vi "ProgrammWithEventAndStateMachine.vi"() -> ()   [LabVIEW 2020]
uses:
  #typedef_States.ctl
  #typedef_Database.ctl
  <vilib>/picture/picture.llb/imagedata.ctl
  <vilib>/event_ctls.llb/eventvkey.ctl
  shell32.dll
panel:
  in  "EndOfProgram":bool
  in  "BROWSEINFO 2":T1={"hWndOwner"=0, "pidlRoot"=0, "pszDisplayName"=0, "lpszTitle"=0, "ulFlags"=1, "lpfn"=0, "lParam"=0, "iImage"=0}
  in  "List of images":i32[](listbox)
  in  "Path":string
  out "2D Picture":picture
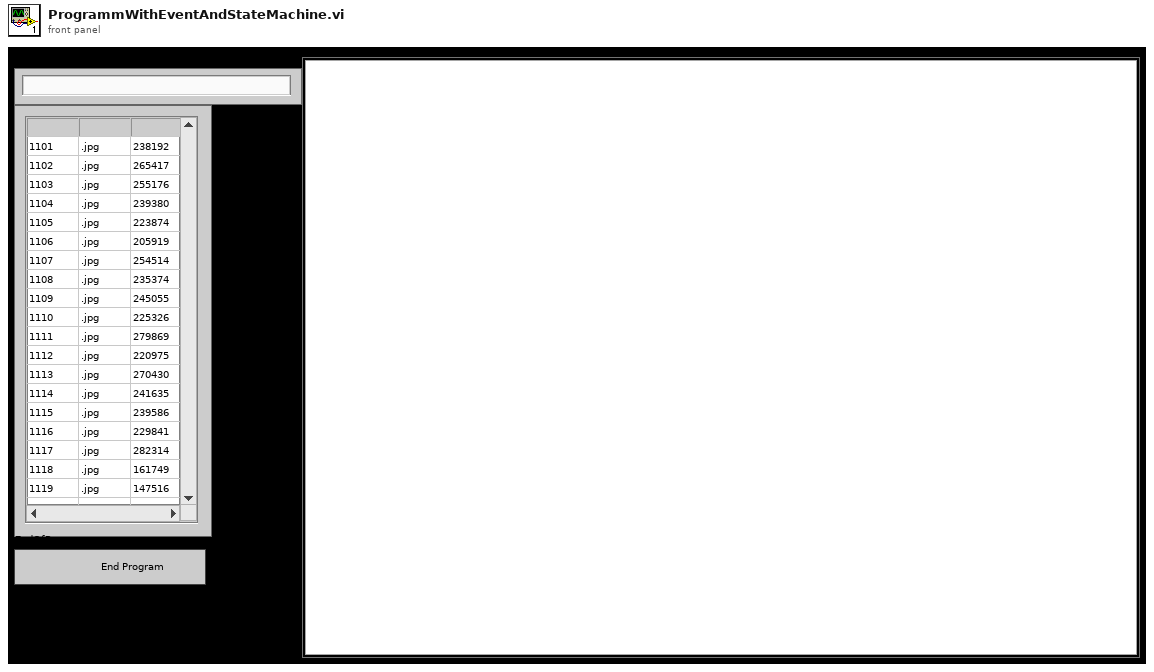
[diagram p1: front panel]
types:
  T1 = cluster{"hWndOwner":i32, "pidlRoot":i32, "pszDisplayName":i32, "lpszTitle":i32, "ulFlags":i32, "lpfn":i32, "lParam":i32, "iImage":i32}
  T2 = typedef "#typedef_States.ctl" = enum16{"Initialize", "CheckButton", "OpenFromKey", "OpenFromPath", "ImageView", "AreaOfImageResize", "ImageResize", "ChangeImage", "ShowNext", "ShowPrevious", "LoadImagesName", "End"}
  T3 = typedef "#typedef_Database.ctl" = cluster{"Folder Directory":string, "Name of images":string[], "PreviousState":T2, "NumberOfRow":i32, "PanelResizeMeasurement":cluster{"Right":i16, "Left":i16, "Bottom":i16, "Top":i16}, "CurrentImageData":T4, "ImageChangeKey":T5, "IsShiftPressed?":bool}
  T4 = typedef "imagedata.ctl" = cluster{"image type":i32, "image depth":i32, "image":u8[], "mask":u8[], "colors":u32[], "Rectangle":cluster{"left":i16, "top":i16, "right":i16, "bottom":i16}}
  T5 = typedef "eventvkey.ctl" = enum16{"ASCII", "Enter", "Return", "Shift", "Ctrl", "Alt", "Cmd", "Opt", "Caps", "NumLock", "Clear", "Break", "Up", "Down", "Left", "Right", "Insert", "Delete", "Home", "End", "PageUp", "PageDown", "Escape", "Help", "Pause", "ScrollLock", "F1", "F2", "F3", "F4", "F5", "F6", "F7", "F8", "F9", "F10", "F11", "F12", "F13", "F14", "F15", "F16", "F17", "F18", "F19", "F20", "F21", "F22", "F23", "F24", "Play", "VolumeUp", "VolumeDown", "Mute", "Two Byte Char"}
  T6 = cluster{"Shift":bool, "Ctrl":bool, "Alt":bool, "Cmd":bool, "Opt":bool}
  T7 = typedef "LVRectTypeDef.ctl" = cluster{"Left":i16, "Top":i16, "Right":i16, "Bottom":i16}
  T8 = typedef "LVBoundsTypeDef.ctl" = cluster{"Width":u32, "Height":u32}
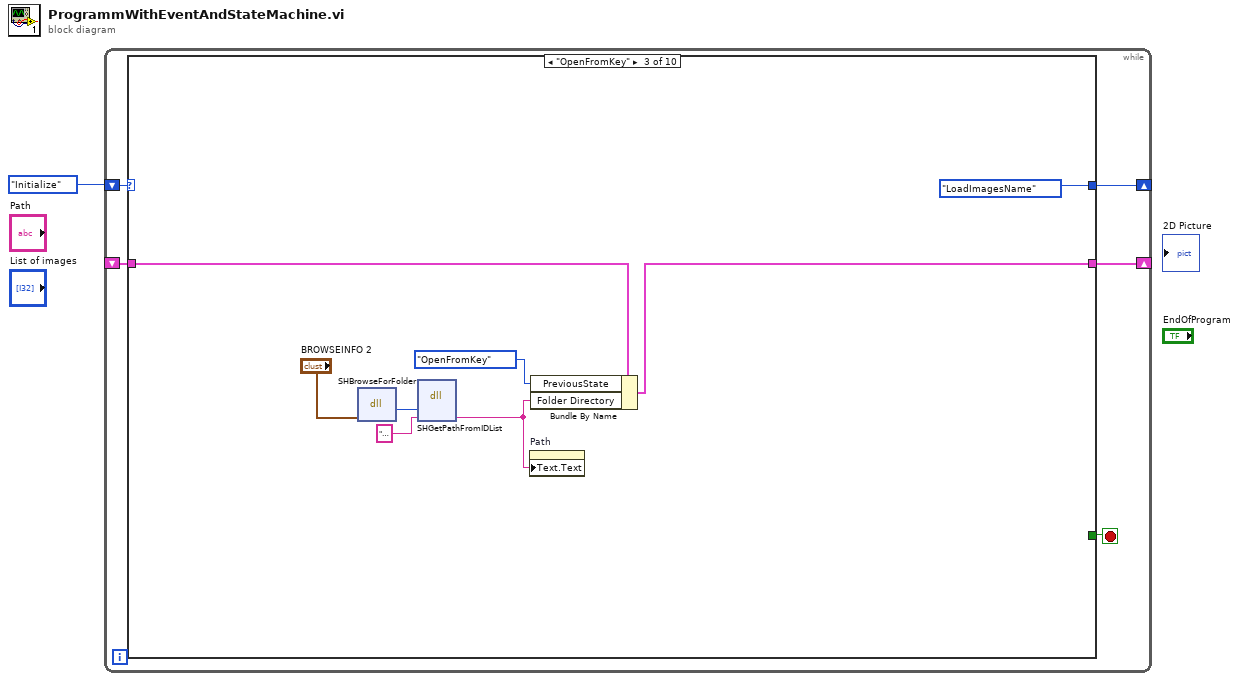
[diagram p0: block diagram]
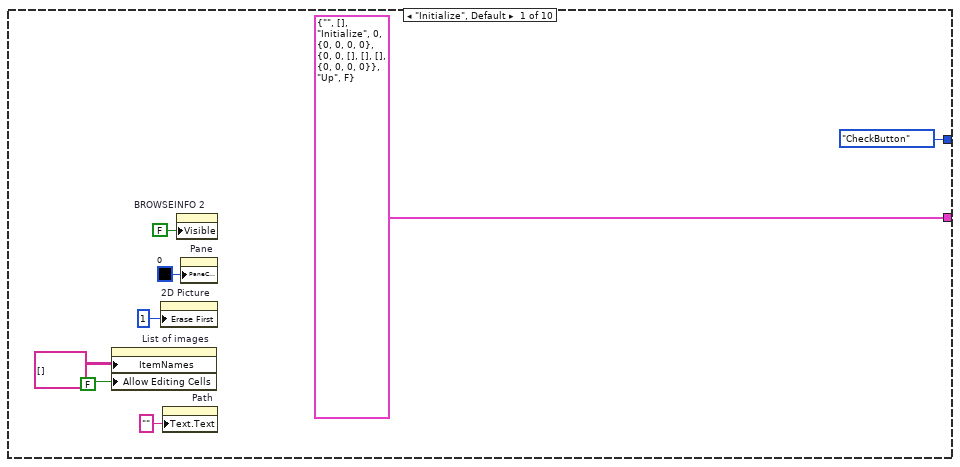
[diagram p2: hidden frame]
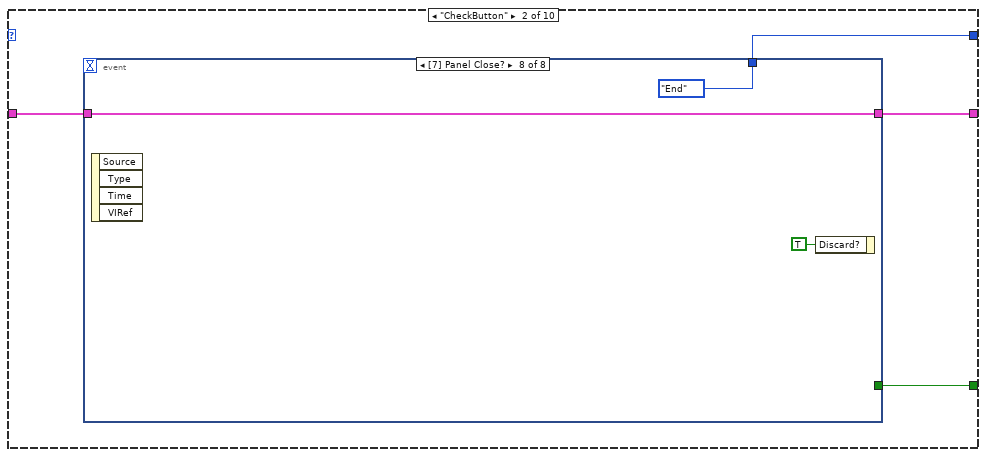
[diagram p3: hidden frame]
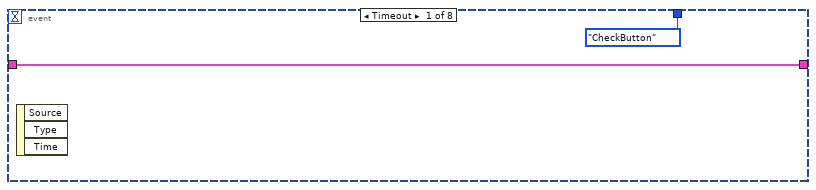
[diagram p4: hidden frame]
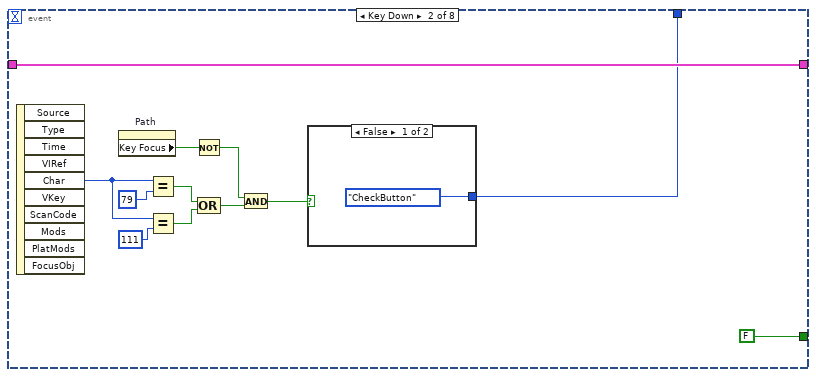
[diagram p5: hidden frame]
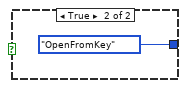
[diagram p6: hidden frame]
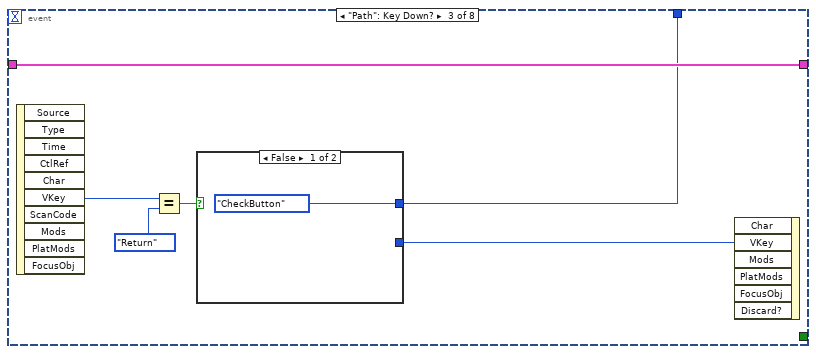
[diagram p7: hidden frame]
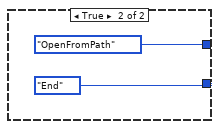
[diagram p8: hidden frame]
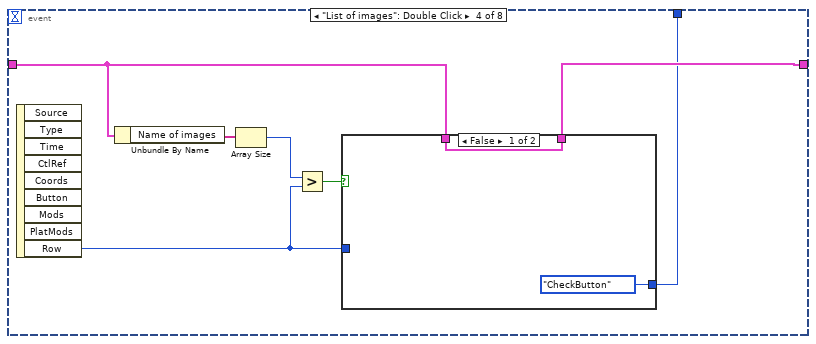
[diagram p9: hidden frame]
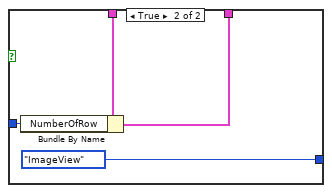
[diagram p10: hidden frame]
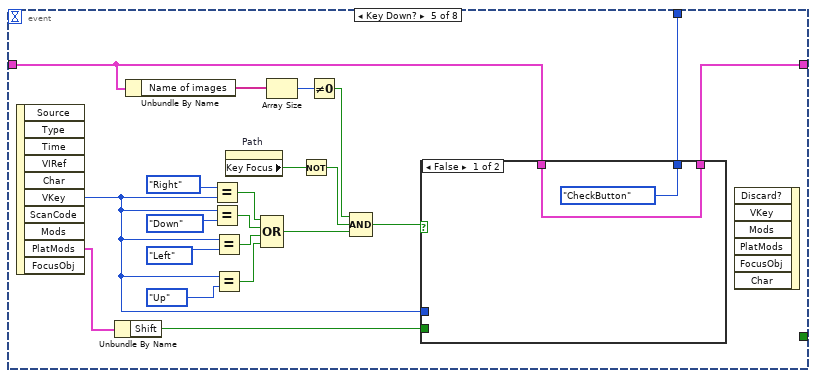
[diagram p11: hidden frame]
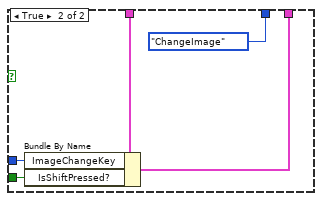
[diagram p12: hidden frame]
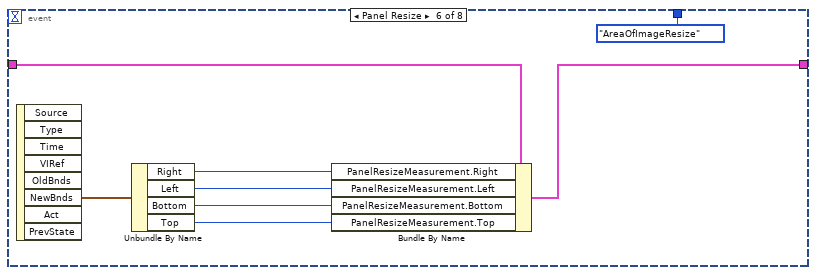
[diagram p13: hidden frame]
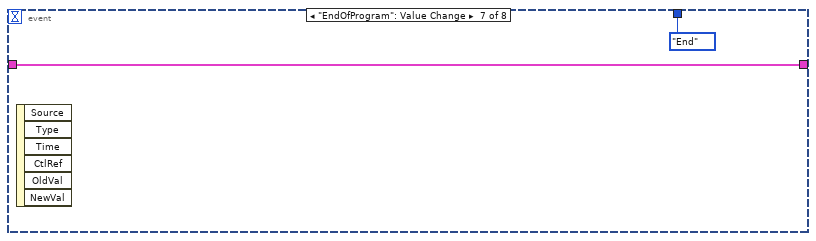
[diagram p14: hidden frame]
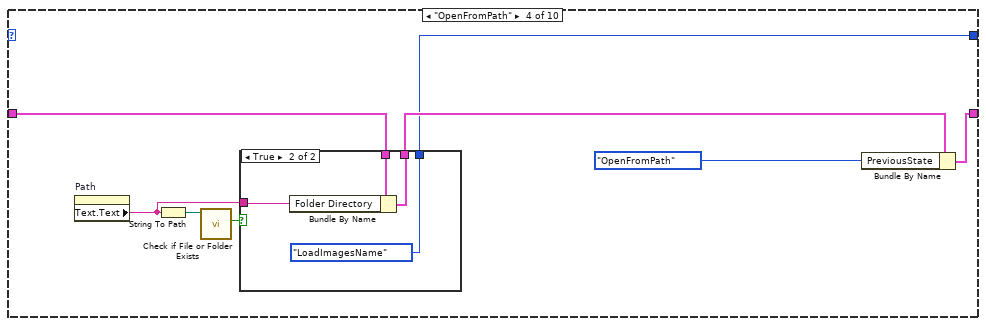
[diagram p15: hidden frame]
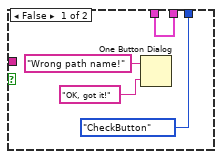
[diagram p16: hidden frame]
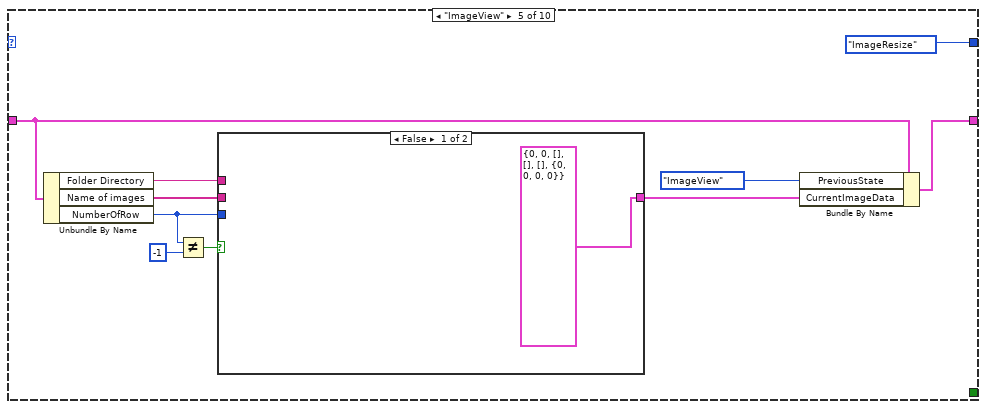
[diagram p17: hidden frame]
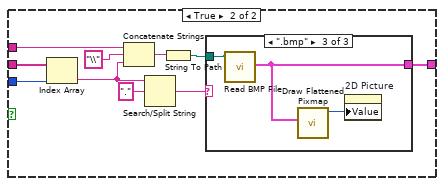
[diagram p18: hidden frame]
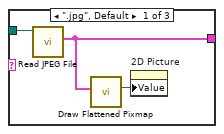
[diagram p19: hidden frame]
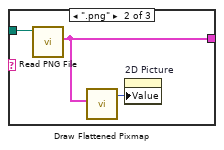
[diagram p20: hidden frame]
diagram:
  n1 = while {
    shift-right: [w2] -> _
    shift-left: _ -> [w6]
    shift-right: [w3] -> _
    shift-left: #typedef_States."Initialize" ("States") -> [w4]
    stop <- w5 stop-if-true
    n2 = case shown="\"OpenFromKey\"" w4 {
      tunnel: w6 -> [_ w18 w102 w110 w128 w155 w176 w181 w252 w273]
      tunnel: [_ w17 _ _ _ _ _ _ _ TRUE] -> w5
      tunnel: [T3 {"Folder Directory"="", "Name of images"=[], "PreviousState"=enum."Initialize", "NumberOfRow"=0, "PanelResizeMeasurement"={"Right"=0, "Left"=0, "Bottom"=0, "Top"=0}, "CurrentImageData"={"image type"=0, "image depth"=0, "image"=[], "mask"=[], "colors"=[], "Rectangle"={"left"=0, "top"=0, "right"=0, "bottom"=0}}, "ImageChangeKey"=enum."Up", "IsShiftPressed?"=FALSE} ("Database") w16 w101 w108 w127 w154 w174 w183 w258 w273] -> w2
      tunnel: [#typedef_States."CheckButton" ("States") w15 #typedef_States."LoadImagesName" ("States") w106 #typedef_States."ImageResize" ("States") #typedef_States."ImageResize" ("States") #typedef_States."CheckButton" ("States") #typedef_States."ImageView" ("States") #typedef_States."ImageView" ("States") #typedef_States."End" ("States")] -> w3
      frame "Initialize", Default {
        n3 = property on="List of images" class="MCListbox (strict)"("ItemNames"=string[][] [] ("Item Names"), "Allow Editing Cells"=FALSE) -> ()  [unwired: 2 in, 2 out]
        n4 = property on="2D Picture" class="Pict"("Erase First"=u8 1) -> ()  [unwired: 2 in, 2 out]
        n5 = property on="Path" class="Str"("Text.Text"="") -> ()  [unwired: 2 in, 2 out]
        n6 = property on="BROWSEINFO 2" class="Clust (strict)"("Visible"=FALSE) -> ()  [unwired: 2 in, 2 out]
        n7 = property on="Pane" class="Pane"("PaneColor"=u32 0 ("Pane Color")) -> ()  [unwired: 2 in, 2 out]
      }
      frame "CheckButton" {
        n8 = event shown="[7] Panel Close?" {
          selector: _ -> [_ _ _ _ _ _ _ _]
          dyn-events: _ -> [_ _ _ _ _ _ _ _]
          timeout: _ -> [_ _ _ _ _ _ _ _]
          tunnel: w18 -> [w20 w22 w36 w49 w65 w91 w94 w95]
          tunnel: [w20 w22 w36 w50 w66 w90 w94 w95] -> w16
          tunnel: [_ FALSE _ _ _ _ _ _] -> w17
          tunnel: [#typedef_States."CheckButton" ("States") w21 w35 w47 w67 #typedef_States."AreaOfImageResize" ("States") #typedef_States."End" ("States") #typedef_States."End" ("States")] -> w15
          event Timeout {
            n9 = event-data() -> ()  [unwired: 1 in, 3 out]
          }
          event Key Down {
            n10 = event-data() -> ("Char"=w32:i16)  [unwired: 1 in, 9 out]
            n11 = property on="Path" class="Str"() -> ("Key Focus"=w26:bool)  [unwired: 2 in, 2 out]
            n12 = Equal?(x=w32, y=i16 79) -> (x = y?=w29:bool)
            n13 = Equal?(x=w32, y=i16 111) -> (x = y?=w28:bool)
            n14 = Not(x=w26) -> (.not. x?=w25:bool)
            n15 = Compound Arithmetic op=OR(w29, w28) -> (w24:bool)
            n16 = And(x=w25, y=w24) -> (x .and. y?=w23:bool)
            n17 = case shown="False" w23 {
              tunnel: [#typedef_States."CheckButton" ("States") #typedef_States."OpenFromKey" ("States")] -> w21
              frame False {
              }
              frame True {
              }
            }
          }
          event "Path": Key Down? {
            n18 = event-data() -> ("VKey"=w39:T5)  [unwired: 1 in, 9 out]
            n19 = Equal?(x=w39, y=eventvkey."Return") -> (x = y?=w40:bool)
            n20 = case shown="False" w40 {
              tunnel: [_ eventvkey."End" ("VKey")] -> w37
              tunnel: [#typedef_States."CheckButton" ("States") #typedef_States."OpenFromPath" ("States")] -> w35
              frame False {
              }
              frame True {
              }
            }
            n21 = event-data("VKey"=w37) -> ()  [unwired: 6 in, 1 out]
          }
          event "List of images": Double Click {
            n22 = event-data() -> ("Row"=w46:i32)  [unwired: 1 in, 8 out]
            n23 = Unbundle By Name(w49) -> ("Name of images"=w48:string[])
            n24 = Array Size(array=w48) -> (size(s)=w44:i32)
            n25 = Greater?(x=w44, y=w46) -> (0:w45:bool)
            n26 = case shown="False" w45 {
              tunnel: w49 -> [w52 w56]
              tunnel: [w52 w55] -> w50
              tunnel: w46 -> [_ w54]
              tunnel: [#typedef_States."CheckButton" ("States") #typedef_States."ImageView" ("States")] -> w47
              frame False {
              }
              frame True {
                n27 = Bundle By Name(cluster=w56, "NumberOfRow"=w54) -> (w55:T3)
              }
            }
          }
          event Key Down? {
            n28 = event-data() -> ("VKey"=w64:T5, "PlatMods"=w58:T6)  [unwired: 1 in, 8 out]
            n29 = Unbundle By Name(w58) -> ("Shift"=w57:bool)
            n30 = Unbundle By Name(w65) -> ("Name of images"=w77:string[])
            n31 = Equal?(x=eventvkey."Right" ("VKey"), y=w64) -> (x = y?=w76:bool)
            n32 = Equal?(x=w64, y=eventvkey."Down" ("VKey")) -> (x = y?=w75:bool)
            n33 = Equal?(x=w64, y=eventvkey."Left" ("VKey")) -> (x = y?=w69:bool)
            n34 = Equal?(x=w64, y=eventvkey."Up" ("VKey")) -> (x = y?=w68:bool)
            n35 = property on="Path" class="Str"() -> ("Key Focus"=w74:bool)  [unwired: 2 in, 2 out]
            n36 = Compound Arithmetic op=OR(w76, w75, w69, w68) -> (w62:bool)
            n37 = Array Size(array=w77) -> (size(s)=w63:i32)
            n38 = Not(x=w74) -> (.not. x?=w61:bool)
            n39 = Not Equal To 0?(x=w63) -> (x != 0?=w60:bool)
            n40 = Compound Arithmetic op=AND(w60, w61, w62) -> (w59:bool)
            n41 = case shown="False" w59 {
              tunnel: [#typedef_States."CheckButton" ("States") #typedef_States."ChangeImage" ("States")] -> w67
              tunnel: w65 -> [w78 w83]
              tunnel: [w78 w82] -> w66
              tunnel: w64 -> [_ w81]
              tunnel: w57 -> [_ w80]
              frame False {
              }
              frame True {
                n42 = Bundle By Name(cluster=w83, "ImageChangeKey"=w81, "IsShiftPressed?"=w80) -> (w82:T3)
              }
            }
            n43 = event-data() -> ()  [unwired: 7 in, 1 out]
          }
          event Panel Resize {
            n44 = event-data() -> ("NewBnds"=w89:T7)  [unwired: 1 in, 7 out]
            n45 = Unbundle By Name(w89) -> ("Right"=w88:i16, "Left"=w87:i16, "Bottom"=w86:i16, "Top"=w85:i16)
            n46 = Bundle By Name(cluster=w91, "PanelResizeMeasurement.Right"=w88, "PanelResizeMeasurement.Left"=w87, "PanelResizeMeasurement.Bottom"=w86, "PanelResizeMeasurement.Top"=w85) -> (w90:T3)
          }
          event "EndOfProgram": Value Change {
            n47 = event-data() -> ()  [unwired: 1 in, 6 out]
          }
          event Panel Close? {
            n48 = event-data() -> ()  [unwired: 1 in, 4 out]
            n49 = event-data("Discard?"=TRUE) -> ()  [unwired: 1 in, 1 out]
          }
        }
      }
      frame "OpenFromKey" {
        n50 = dll-call lib="shell32.dll" fn="SHBrowseForFolder"("BROWSEINFO"="BROWSEINFO 2") -> ("PointerToIDList"=w104:i32)  [unwired: 4 in, 2 out]
        n51 = dll-call lib="shell32.dll" fn="SHGetPathFromIDList"("PointerToIDList"=w104, "PathBuffer"="                                                                                                                                                                                                                                                                    " ("260 char string")) -> ("PathBuffer"=w98:string)  [unwired: 5 in, 2 out]
        n52 = property on="Path" class="Str"("Text.Text"=w98) -> ()  [unwired: 2 in, 2 out]
        n53 = Bundle By Name(cluster=w102, "PreviousState"=#typedef_States."OpenFromKey" ("States"), "Folder Directory"=w98) -> (w101:T3)
      }
      frame "OpenFromPath" {
        n54 = property on="Path" class="Str"() -> ("Text.Text"=w111:string)  [unwired: 2 in, 2 out]
        n55 = String To Path(string=w111) -> (path=w113:path)
        n56 = call <vilib>:"Check if File or Folder Exists.vi"("path"=w113) -> ("file or folder exists?"=w112:bool)  [unwired: 8 in, 2 out]
        n57 = case shown="True" w112 {
          tunnel: w110 -> [w117 w121]
          tunnel: w111 -> [_ w119]
          tunnel: [w117 w120] -> w109
          tunnel: [#typedef_States."CheckButton" ("States") #typedef_States."LoadImagesName" ("States")] -> w106
          frame False {
            n58 = One Button Dialog(message="Wrong path name!", button name ("OK")="OK, got it!") -> ()  [unwired: 1 out]
          }
          frame True {
            n59 = Bundle By Name(cluster=w121, "Folder Directory"=w119) -> (w120:T3)
          }
        }
        n60 = Bundle By Name(cluster=w109, "PreviousState"=#typedef_States."OpenFromPath" ("States")) -> (w108:T3)
      }
      frame "ImageView" {
        n61 = Unbundle By Name(w128) -> ("Folder Directory"=w130:string, "Name of images"=w131:string[], "NumberOfRow"=w123:i32)
        n62 = Not Equal?(x=w123, y=-1) -> (x != y?=w124:bool)
        n63 = case shown="False" w124 {
          tunnel: w131 -> [_ w142]
          tunnel: w130 -> [_ w141]
          tunnel: w123 -> [_ w134]
          tunnel: [T4 {"image type"=0, "image depth"=0, "image"=[], "mask"=[], "colors"=[], "Rectangle"={"left"=0, "top"=0, "right"=0, "bottom"=0}} ("CurrentImageData") w133] -> w125
          frame False {
          }
          frame True {
            n64 = Index Array(array=w142, index=w134) -> (element=w139:string)
            n65 = Concatenate Strings(w141, "\\" ("string"), w139) -> (w140:string)
            n66 = Search/Split String(string=w139, search string/char (-)=".") -> (match + rest of string=w138:string)  [unwired: 1 in, 2 out]
            n67 = String To Path(string=w140) -> (path=w137:path)
            n68 = case shown="\".bmp\"" w138 {
              tunnel: w137 -> [w145 w147 w150]
              tunnel: [w143 w146 w149] -> w133
              frame ".jpg", Default {
                n69 = call <vilib>:"Read JPEG File.vi"("path to JPEG file"=w145) -> ("image data"=w143:T4)  [unwired: 8 in, 2 out]
                n70 = call <vilib>:"Draw Flattened Pixmap.vi"("image data"=w143) -> ("new picture"=w144:picture)  [unwired: 8 in]
                n71 = property on="2D Picture" class="Pict"("Value"=w144) -> ()  [unwired: 2 in, 2 out]
              }
              frame ".png" {
                n72 = call <vilib>:"Read PNG File.vi"("path to PNG file"=w147) -> ("image data"=w146:T4)  [unwired: 8 in, 2 out]
                n73 = call <vilib>:"Draw Flattened Pixmap.vi"("image data"=w146) -> ("new picture"=w148:picture)  [unwired: 8 in]
                n74 = property on="2D Picture" class="Pict"("Value"=w148) -> ()  [unwired: 2 in, 2 out]
              }
              frame ".bmp" {
                n75 = call <vilib>:"Read BMP File.vi"("path to BMP file"=w150) -> ("image data"=w149:T4)  [unwired: 8 in, 2 out]
                n76 = call <vilib>:"Draw Flattened Pixmap.vi"("image data"=w149) -> ("new picture"=w151:picture)  [unwired: 8 in]
                n77 = property on="2D Picture" class="Pict"("Value"=w151) -> ()  [unwired: 2 in, 2 out]
              }
            }
          }
        }
        n78 = Bundle By Name(cluster=w128, "PreviousState"=#typedef_States."ImageView" ("States"), "CurrentImageData"=w125) -> (w127:T3)
      }
      frame "AreaOfImageResize" {
        n79 = Unbundle By Name(w155) -> ("PanelResizeMeasurement.Right"=w159:i16, "PanelResizeMeasurement.Left"=w158:i16, "PanelResizeMeasurement.Bottom"=w157:i16, "PanelResizeMeasurement.Top"=w156:i16)
        n80 = Subtract(x=w159, y=w158) -> (x-y=w172:i16)
        n81 = Subtract(x=w157, y=w156) -> (x-y=w171:i16)
        n82 = property on="Path" class="Str"() -> ("Width"=w166:u32)  [unwired: 2 in, 2 out]
        n83 = To Word Integer(number=w166) -> (16bit integer=w163:i16)
        n84 = Subtract(x=w171, y=i16 5) -> (x-y=w168:i16)
        n85 = To Unsigned Long Integer(number=w168) -> (unsigned 32bit integer=w164:u32)
        n86 = Add(x=w163, y=i16 30) -> (x+y=w162:i16)
        n87 = property on="2D Picture" class="Pict"() -> ("Draw Area Size"=w170:T8)  [unwired: 2 in, 2 out]
        n88 = Subtract(x=w172, y=w162) -> (x-y=w169:i16)
        n89 = To Unsigned Long Integer(number=w169) -> (unsigned 32bit integer=w165:u32)
        n90 = Bundle By Name(cluster=w170, "Width"=w165, "Height"=w164) -> (w167:T8)
        n91 = property on="2D Picture" class="Pict"("Draw Area Size"=w167) -> ()  [unwired: 2 in, 2 out]
        n92 = Bundle By Name(cluster=w155, "PreviousState"=#typedef_States."AreaOfImageResize" ("States")) -> (w154:T3)
      }
      frame "ImageResize" {
        n93 = Unbundle By Name(w176) -> ("CurrentImageData"=w177:T4)
        n94 = control-ref of="2D Picture"() -> (w178:refnum<vi>)
        n95 = call "PictureAdjust.vi"("image data"=w177, "Picture in"=w178) -> ("Numeric"=w179:dbl)  [unwired: 9 in]
        n96 = property on="2D Picture" class="Pict"("ZoomFactor"=w179) -> ()  [unwired: 2 in, 2 out]
        n97 = Bundle By Name(cluster=w176, "PreviousState"=#typedef_States."ImageResize" ("States")) -> (w174:T3)
      }
      frame "ChangeImage" {
        n98 = Unbundle By Name(w181) -> ("IsShiftPressed?"=w180:bool)
        n99 = case shown="False" w180 {
          tunnel: w181 -> [w187 w224]
          tunnel: [w186 w223] -> w184
          frame False {
            n100 = Unbundle By Name(w187) -> ("ImageChangeKey"=w192:T5)
            n101 = Equal?(x=eventvkey."Right" ("ImageChangeKey"), y=w192) -> (x = y?=w190:bool)
            n102 = Equal?(x=w192, y=eventvkey."Down" ("ImageChangeKey")) -> (x = y?=w189:bool)
            n103 = Compound Arithmetic op=OR(w190, w189) -> (w188:bool)
            n104 = case shown="False" w188 {
              tunnel: w187 -> [w197 w211]
              tunnel: [w196 w209] -> w186
              frame False {
                n105 = Unbundle By Name(w197) -> ("NumberOfRow"=w195:i32, "Name of images"=w194:string[])
                n106 = Greater?(x=w195, y=0) -> (0:w198:bool)
                n107 = case shown="False" w198 {
                  tunnel: w197 -> [w204 w208]
                  tunnel: [w203 w207] -> w196
                  tunnel: w195 -> [_ w206]
                  tunnel: w194 -> [w201 _]
                  frame False {
                    n108 = Array Size(array=w201) -> (size(s)=w202:i32)
                    n109 = Decrement(x=w202) -> (x-1=w200:i32)
                    n110 = Bundle By Name(cluster=w204, "NumberOfRow"=w200) -> (w203:T3)
                  }
                  frame True {
                    n111 = Decrement(x=w206) -> (x-1=w205:i32)
                    n112 = Bundle By Name(cluster=w208, "NumberOfRow"=w205) -> (w207:T3)
                  }
                }
              }
              frame True {
                n113 = Unbundle By Name(w211) -> ("NumberOfRow"=w210:i32, "Name of images"=w214:string[])
                n114 = Array Size(array=w214) -> (size(s)=w213:i32)
                n115 = Decrement(x=w213) -> (x-1=w212:i32)
                n116 = Less?(x=w210, y=w212) -> (x < y?=w215:bool)
                n117 = case shown="True" w215 {
                  tunnel: w211 -> [w218 w222]
                  tunnel: w210 -> [_ w221]
                  tunnel: [w217 w219] -> w209
                  frame False {
                    n118 = Bundle By Name(cluster=w218, "NumberOfRow"=0) -> (w217:T3)
                  }
                  frame True {
                    n119 = Increment(x=w221) -> (x+1=w220:i32)
                    n120 = Bundle By Name(cluster=w222, "NumberOfRow"=w220) -> (w219:T3)
                  }
                }
              }
            }
          }
          frame True {
            n121 = Unbundle By Name(w224) -> ("ImageChangeKey"=w229:T5)
            n122 = Equal?(x=eventvkey."Right" ("ImageChangeKey"), y=w229) -> (x = y?=w227:bool)
            n123 = Equal?(x=w229, y=eventvkey."Down" ("ImageChangeKey")) -> (x = y?=w226:bool)
            n124 = Compound Arithmetic op=OR(w227, w226) -> (w225:bool)
            n125 = case shown="True" w225 {
              tunnel: w224 -> [w232 w243]
              tunnel: [w231 w242] -> w223
              frame False {
                n126 = Unbundle By Name(w232) -> ("Name of images"=w240:string[], "NumberOfRow"=w234:i32)
                n127 = Array Size(array=w240) -> (size(s)=w239:i32)
                n128 = Subtract(x=w234, y=10) -> (x-y=w233:i32)
                n129 = Decrement(x=w239) -> (x-1=w238:i32)
                n130 = In Range and Coerce(upper limit=w238, x=w233, lower limit=0) -> (coerced(x)=w236:i32)  [unwired: 1 out]
                n131 = Bundle By Name(cluster=w232, "NumberOfRow"=w236) -> (w231:T3)
              }
              frame True {
                n132 = Unbundle By Name(w243) -> ("Name of images"=w250:string[], "NumberOfRow"=w248:i32)
                n133 = Array Size(array=w250) -> (size(s)=w249:i32)
                n134 = Add(x=w248, y=10) -> (x+y=w245:i32)
                n135 = Decrement(x=w249) -> (x-1=w246:i32)
                n136 = In Range and Coerce(upper limit=w246, x=w245, lower limit=0) -> (coerced(x)=w241:i32)  [unwired: 1 out]
                n137 = Bundle By Name(cluster=w243, "NumberOfRow"=w241) -> (w242:T3)
              }
            }
          }
        }
        n138 = Bundle By Name(cluster=w184, "PreviousState"=#typedef_States."ChangeImage" ("States")) -> (w183:T3)
      }
      frame "LoadImagesName" {
        n139 = Unbundle By Name(w252) -> ("Folder Directory"=w261:string)
        n140 = String To Path(string=w261) -> (path=w263:path)
        n141 = for {
          tunnel: w263 -> [w272]
          tunnel: [w270] -> w256 mode=concatenating
          tunnel: string[] ["*.bmp", "*.jpg", "*.png"] -> [w271] mode=indexing
          n142 = List Folder(path=w272, pattern=w271) -> (filenames=w270:string[])  [unwired: 2 in, 3 out]
        }
        n143 = call "ListofImages(name,ext,size).vi"("Folder Directory"=w261, "Name of images"=w256) -> ("List of images (name, ext, size)"=w260:string[][])  [unwired: 9 in]
        n144 = Array Size(array=w256) -> (size(s)=w255:i32)
        n145 = property on="List of images" class="MCListbox (strict)"("ItemNames"=w260, "NumCols"=u32 3 ("Number of Columns")) -> ()  [unwired: 2 in, 2 out]
        n146 = Greater Than 0?(x=w255) -> (x > 0?=w254:bool)
        n147 = case shown="False" w254 {
          tunnel: w252 -> [w265 w269]
          tunnel: [w264 w268] -> w253
          frame False {
            n148 = Bundle By Name(cluster=w265, "NumberOfRow"=-1) -> (w264:T3)
          }
          frame True {
            n149 = Bundle By Name(cluster=w269, "NumberOfRow"=0) -> (w268:T3)
          }
        }
        n150 = Bundle By Name(cluster=w253, "Name of images"=w256, "PreviousState"=#typedef_States."LoadImagesName" ("States")) -> (w258:T3)
      }
      frame "End" {
      }
    }
  }
